vi "Launch Nested Actors.vi"(8 "error in (no error)":errorcluster, 11 "Turbo in":refnum<class "Turbo.lvclass">) -> (0 "error out":errorcluster, 3 "Turbo out":refnum<class "Turbo.lvclass">)   [LabVIEW 2015, in "cRIO-Carbondioxide.lvlib" / "CO2-Actor.lvlib" / "Turbo.lvclass"]
uses:
  Turbo.lvclass
  <vilib>/ActorFramework/Actor/Actor.lvclass
  Valve/Action.ctl
  Turbo.lvclass/Turbo.ctl
  CO2 Actor/CO2 Actor.lvclass
  Valve/Valve.lvclass
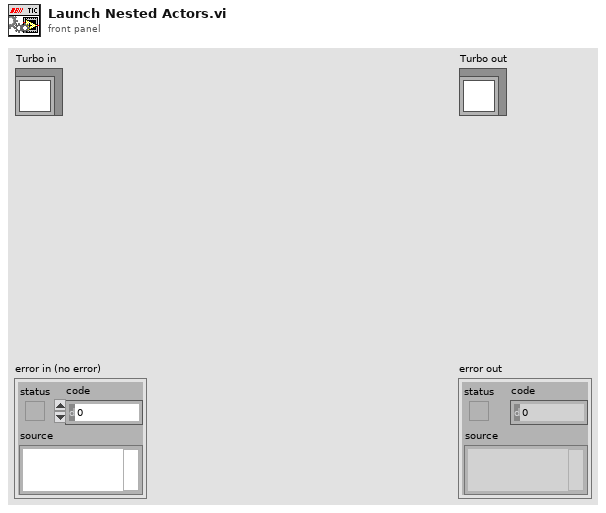
[diagram p1: front panel]
types:
  T1 = typedef "Action.ctl" = enum16{"Open", "Close", "None"}
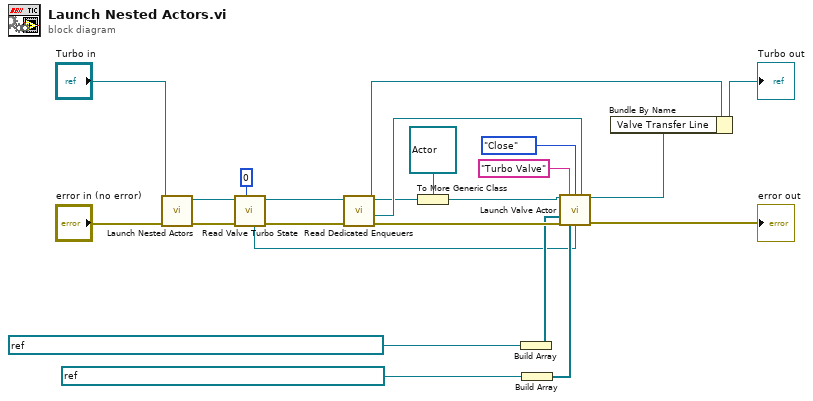
[diagram p0: block diagram]
diagram:
  n1 = call-parent "Launch Nested Actors.vi"("error in (no error)"="error in (no error)", "CO2 Actor in"="Turbo in") -> ("error out"=w6:errorcluster, "CO2 Actor out"=w4:refnum<class "Turbo.lvclass">)  [unwired: 8 in]
  n2 = call "Read Valve Turbo State.vi"("timeout in ms (-1)"=0, "error in (no error)"=w6, "Turbo in"=w4) -> ("error out"=w5:errorcluster, "Turbo out"=w7:refnum<class "Turbo.lvclass">, "Valve Turbo StateQ"=w2:refnum<queue>)  [unwired: 5 in, 1 out]
  n3 = call "Read Dedicated Enqueuers.vi"("error in (no error)"=w5, "CO2 Actor in"=w7) -> ("error out"=w18:errorcluster, "DedicatedEnQrs"=w16:refnum<queue>, "CO2 Actor out"=w3:refnum<class "Turbo.lvclass">)  [unwired: 6 in, 1 out]
  n4 = To More Generic Class(target class=refnum<class "Actor.lvclass"> refnum ("Caller Actor in"), reference=w3) -> (generic class reference=w19:refnum<class "Actor.lvclass">)
  n5 = Build Array(refnum<k21> "ni.var.psp://crio-carbondioxide/AMS Gas SHV/Valves/Turbo Valve" ("SHV")) -> (w9:refnum<k21>[])
  n6 = Build Array(refnum<k21> "ni.var.io://crio-carbondioxide/Mod2/Turbo Valve DV313" ("SHV")) -> (w8:refnum<k21>[])
  n7 = call "Launch Valve Actor.vi"("Caller Actor in"=w19, "Name"="Turbo Valve", "Start Action (Open)"=Action."Close", "DedicatedEnQrs"=w16, "SHV Aliases"=w9, "error in (no error)"=w18, "SHV"=w8, "StateQ"=w2) -> ("Caller-To-Actor Enqueuer"=w14:refnum<class "Message Enqueuer.lvclass">, "error out"=→"error out":errorcluster)  [unwired: 6 in]
  n8 = Bundle By Name(cluster=w3, "Valve Transfer Line"=w14) -> (→"Turbo out":refnum<class "Turbo.lvclass">)
